vi "Get Line Name.vi"(8 "error in":errorcluster, 11 "Line in":T1) -> (0 "error out":errorcluster, 2 "Name":string, 3 "Line out":T1)   [LabVIEW 2015, in "Sequencer Module configuration.lvclass"]
doc: "This VI retrieves the line name or ID, that identifies this element in the cluster, from the line."
uses:
  Sequencer Module configuration.lvclass
  Line.ctl
  classes/Sequence Config/Sequence Config.lvclass
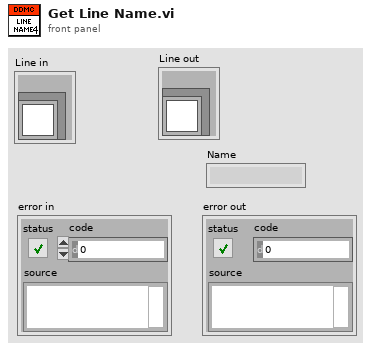
[diagram p1: front panel]
types:
  T1 = typedef "Sequencer Module configuration.lvclass/Line.ctl" = cluster{"Sequence":refnum<class "Sequence Config.lvclass">}
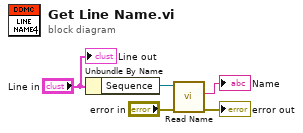
[diagram p0: block diagram]
diagram:
  n1 = Unbundle By Name("Line in") -> ("Sequence"=w4:refnum<class "Sequence Config.lvclass">)
  n2 = call-dynamic "Read Name.vi"("error in (no error)"="error in", "Sequence in"=w4) -> ("error out"=→"error out":errorcluster, "Name"=→"Name":string)  [unwired: 7 in, 1 out]
  "Line out" <- "Line in"
